vi "Close.vi"(8 "error in (no error)":errorcluster, 11 "VI Probe in":refnum<class "PL MKS VI Probe.lvclass">) -> (0 "error out":errorcluster)   [LabVIEW 2015, in "PL MKS VI Probe.lvclass"]
doc: "Closes connection to device."
uses:
  PL MKS VI Probe.lvclass
  PL MKS VI Probe.lvclass/PL MKS VI Probe.ctl
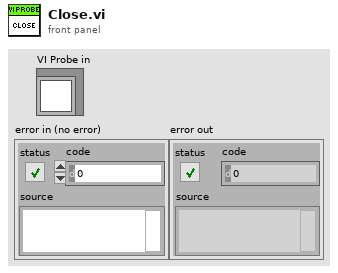
[diagram p1: front panel]
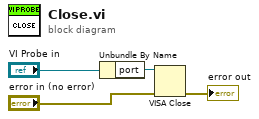
[diagram p0: block diagram]
diagram:
  n1 = Unbundle By Name("VI Probe in") -> ("port"=w3:refnum<visa-resource-name>)
  n2 = VISA Close(VISA resource name=w3, error in (no error)="error in (no error)") -> (error out=→"error out":errorcluster)
